vi "Unpack Imaging Data Control.vi"(9 "Output ready":bool, 10 "input valid":bool, 11 "Data":T1) -> (1 "Input ready":bool, 2 "output valid?":bool, 3 "Unpacked data":u32)   [LabVIEW 2015]
uses:
  OpenScan Labview code_20170126/DRAM data index.ctl
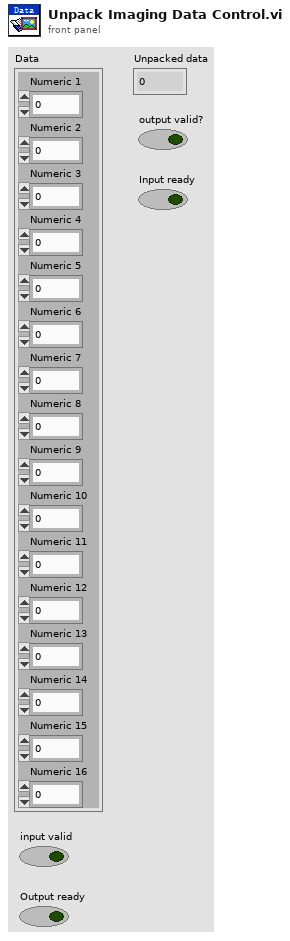
[diagram p1: front panel]
types:
  T1 = cluster{"Numeric 1":u32, "Numeric 2":u32, "Numeric 3":u32, "Numeric 4":u32, "Numeric 5":u32, "Numeric 6":u32, "Numeric 7":u32, "Numeric 8":u32, "Numeric 9":u32, "Numeric 10":u32, "Numeric 11":u32, "Numeric 12":u32, "Numeric 13":u32, "Numeric 14":u32, "Numeric 15":u32, "Numeric 16":u32}
  T2 = typedef "DRAM data index.ctl" = enum16{"Numeric 1", "Numeric 2", "Numeric 3", "Numeric 4", "Numeric 5", "Numeric 6", "Numeric 7", "Numeric 8", "Numeric 9", "Numeric 10", "Numeric 11", "Numeric 12", "Numeric 13", "Numeric 14", "Numeric 15", "Numeric 16"}
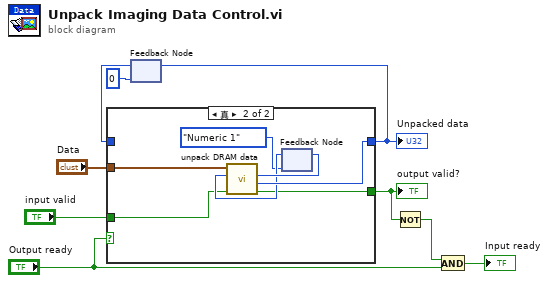
[diagram p0: block diagram]
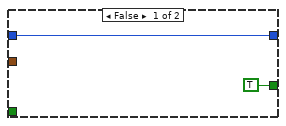
[diagram p2: hidden frame]
diagram:
  n1 = feedback #1(u32 0 ("Unpacked data")) -> (w7:u32)
  n2 = case shown="真" "Output ready" {
    tunnel: "Data" -> [_ w18]
    tunnel: [w11 w17] -> w8
    tunnel: [TRUE ("output valid?") w13] -> w2
    tunnel: "input valid" -> [_ w12]
    tunnel: w7 -> [w11 _]
    frame False {
    }
    frame True {
      n3 = feedback #2(DRAM_data_index."Numeric 1" ("DRAM pack index out")) -> (w15:T2)
      n4 = call "unpack DRAM data.vi"("input valid?"=w12, "DRAM pack index in"=w15, "packer in"=w18) -> ("output valid?"=w13:bool, "Unpacked data"=w17:u32, "DRAM pack index out"=w16:T2)  [unwired: 5 in, 1 out]
      n5 = feedback-in #2(w16) -> ()
    }
  }
  "Unpacked data" <- w8
  "output valid?" <- w2
  n6 = feedback-in #1(w8) -> ()
  n7 = Not(x=w2) -> (.not. x?=w3:bool)
  n8 = And(x=w3, y="Output ready") -> (x .and. y?=→"Input ready":bool)
